vi "init data maps.vi"(11 "input cluster":T4) -> (3 "Data Maps Out":T1[](array[typedef]))   [LabVIEW 2014, in "SQLite runtime.lvclass"]
uses:
  SQLite runtime.lvclass
  <vilib>/NI/Tag Bus/dictionary/full data dictionary.ctl
  data map.ctl
  <vilib>/NI/Tag Bus/tag/Data Type.ctl
  sqlite type.ctl
  <vilib>/NI/Tag Bus/tag/tag descriptor.lvclass
  <vilib>/NI/Tag Bus/dictionary/data dictionary.lvclass
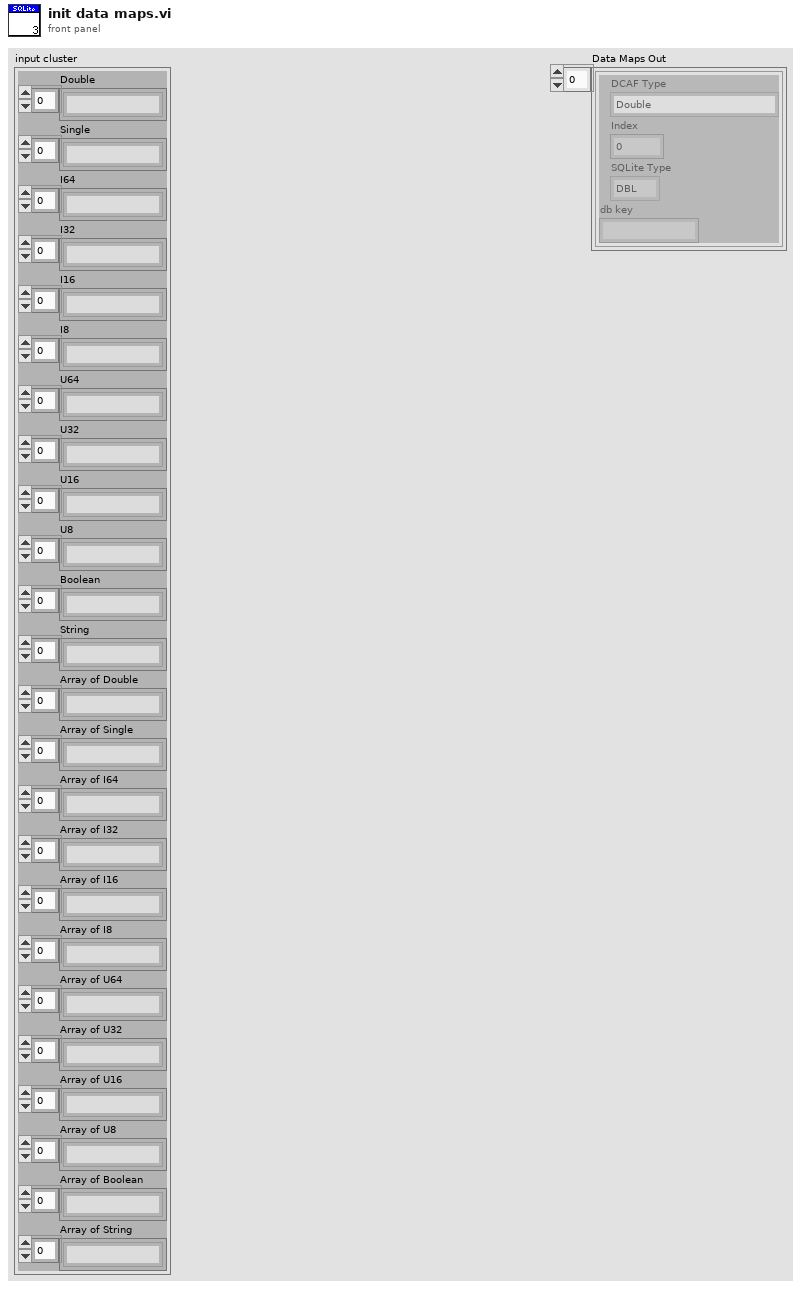
[diagram p1: front panel]
types:
  T1 = typedef "SQLite runtime.lvclass/data map.ctl" = cluster{"DCAF Type":T2, "Index":i32, "SQLite Type":T3, "db key":string}
  T2 = typedef "tag bus.lvlib/tag descriptor.lvclass/Data Type.ctl" = enum16{"Double", "Single", "I64", "I32", "I16", "I8", "U64", "U32", "U16", "U8", "Boolean", "String", "Array of Double", "Array of Single", "Array of I64", "Array of I32", "Array of I16", "Array of I8", "Array of U64", "Array of U32", "Array of U16", "Array of U8", "Array of Boolean", "Array of String"}
  T3 = typedef "SQLite runtime.lvclass/sqlite type.ctl" = enum16{"DBL", "I64", "String"}
  T4 = typedef "tag bus.lvlib/data dictionary.lvclass/full data dictionary.ctl" = cluster{"Double":string[], "Single":string[], "I64":string[], "I32":string[], "I16":string[], "I8":string[], "U64":string[], "U32":string[], "U16":string[], "U8":string[], "Boolean":string[], "String":string[], "Array of Double":string[], "Array of Single":string[], "Array of I64":string[], "Array of I32":string[], "Array of I16":string[], "Array of I8":string[], "Array of U64":string[], "Array of U32":string[], "Array of U16":string[], "Array of U8":string[], "Array of Boolean":string[], "Array of String":string[]}
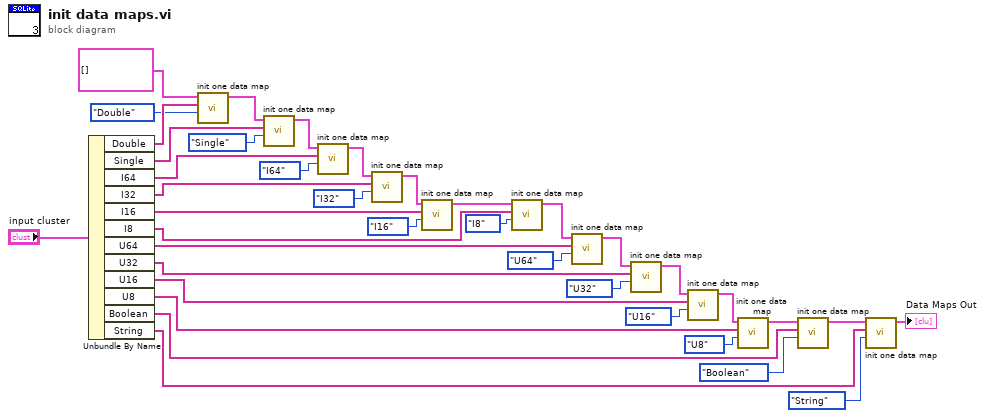
[diagram p0: block diagram]
diagram:
  n1 = Unbundle By Name("input cluster") -> ("Double"=w36:string[], "Single"=w34:string[], "I64"=w32:string[], "I32"=w30:string[], "I16"=w28:string[], "I8"=w26:string[], "U64"=w24:string[], "U32"=w22:string[], "U16"=w20:string[], "U8"=w18:string[], "Boolean"=w16:string[], "String"=w14:string[])
  n2 = call "init one data map.vi"("DCAF Type"=Data_Type."Double", "Allocations"=w36, "Data Maps In"=T1[] []) -> ("Data Maps Out"=w35:T1[])  [unwired: 8 in]
  n3 = call "init one data map.vi"("DCAF Type"=Data_Type."Single", "Allocations"=w34, "Data Maps In"=w35) -> ("Data Maps Out"=w33:T1[])  [unwired: 8 in]
  n4 = call "init one data map.vi"("DCAF Type"=Data_Type."I64", "Allocations"=w32, "Data Maps In"=w33) -> ("Data Maps Out"=w31:T1[])  [unwired: 8 in]
  n5 = call "init one data map.vi"("DCAF Type"=Data_Type."I32", "Allocations"=w30, "Data Maps In"=w31) -> ("Data Maps Out"=w29:T1[])  [unwired: 8 in]
  n6 = call "init one data map.vi"("DCAF Type"=Data_Type."I16", "Allocations"=w28, "Data Maps In"=w29) -> ("Data Maps Out"=w27:T1[])  [unwired: 8 in]
  n7 = call "init one data map.vi"("DCAF Type"=Data_Type."I8", "Allocations"=w26, "Data Maps In"=w27) -> ("Data Maps Out"=w25:T1[])  [unwired: 8 in]
  n8 = call "init one data map.vi"("DCAF Type"=Data_Type."U64", "Allocations"=w24, "Data Maps In"=w25) -> ("Data Maps Out"=w23:T1[])  [unwired: 8 in]
  n9 = call "init one data map.vi"("DCAF Type"=Data_Type."U32", "Allocations"=w22, "Data Maps In"=w23) -> ("Data Maps Out"=w21:T1[])  [unwired: 8 in]
  n10 = call "init one data map.vi"("DCAF Type"=Data_Type."U16", "Allocations"=w20, "Data Maps In"=w21) -> ("Data Maps Out"=w19:T1[])  [unwired: 8 in]
  n11 = call "init one data map.vi"("DCAF Type"=Data_Type."U8", "Allocations"=w18, "Data Maps In"=w19) -> ("Data Maps Out"=w17:T1[])  [unwired: 8 in]
  n12 = call "init one data map.vi"("DCAF Type"=Data_Type."Boolean", "Allocations"=w16, "Data Maps In"=w17) -> ("Data Maps Out"=w15:T1[])  [unwired: 8 in]
  n13 = call "init one data map.vi"("DCAF Type"=Data_Type."String", "Allocations"=w14, "Data Maps In"=w15) -> ("Data Maps Out"=→"Data Maps Out":T1[])  [unwired: 8 in]
